vi "nipkg-updateControlFileMetadataField.vi"(0 "Package data":T1, 5 "Metadata field name":string, 7 "Metadata field index":u8, 9 "Metadata field value":string, 11 "error in (no error)":errorcluster) -> (4 "Package data out":T1, 15 "error out":errorcluster)   [LabVIEW 2014, in "nipkg-build-system.lvlib"]
uses:
  nipkg-build-system.lvlib
  types/Package data.ctl
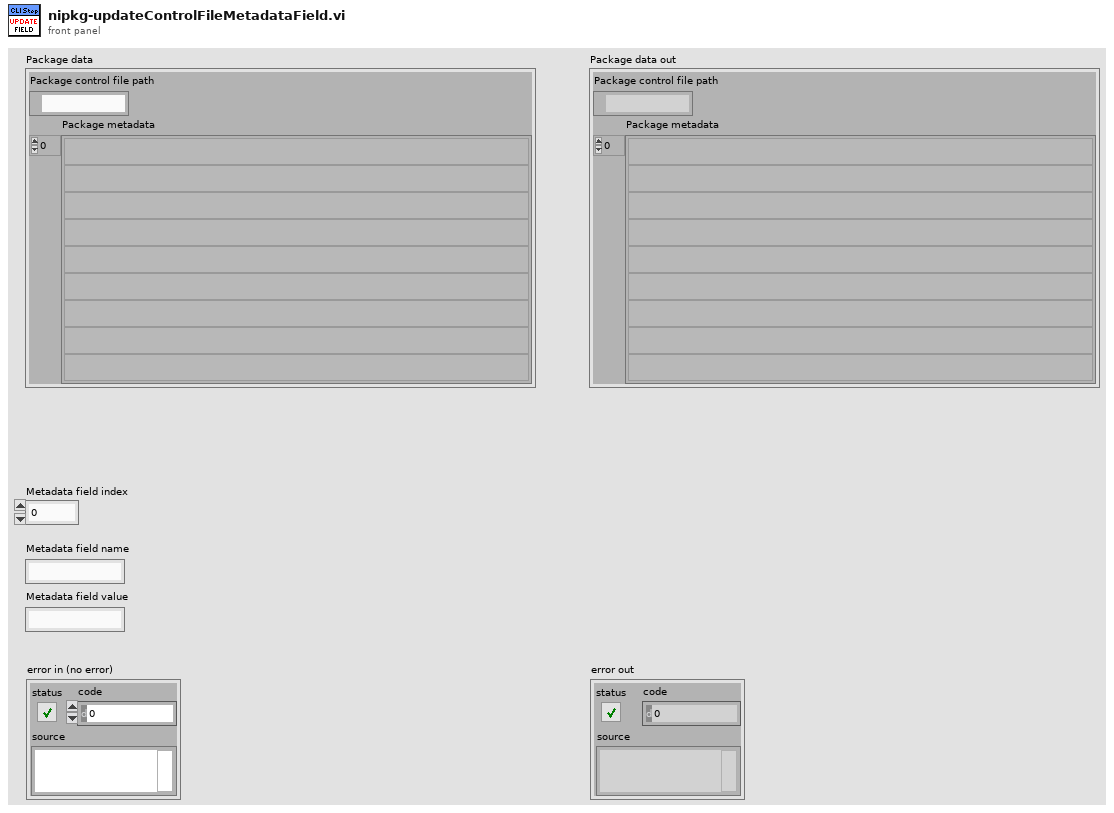
[diagram p1: front panel]
types:
  T1 = typedef "nipkg-build-system.lvlib/Package data.ctl" = cluster{"Package control file path":path, "Package metadata":string[]}
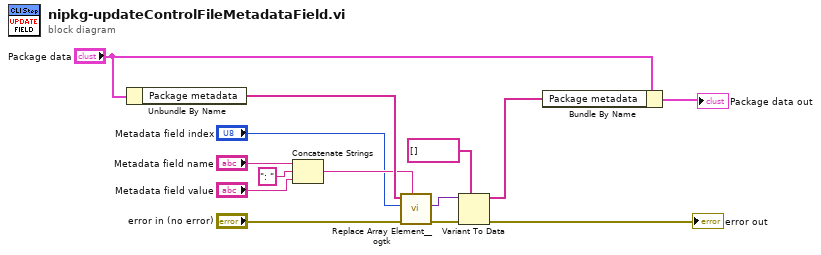
[diagram p0: block diagram]
diagram:
  n1 = Unbundle By Name("Package data") -> ("Package metadata"=w11:string[])
  n2 = Concatenate Strings("Metadata field name", ": " ("string"), "Metadata field value") -> (w10:string)
  n3 = call <userlib>:"Replace Array Element__ogtk.vi"("New Element"=w10, "error in (no error)"="error in (no error)", "Index (1D)"="Metadata field index", "MultiD Array"=w11) -> ("error out"=w6:errorcluster, "VMultiD Array"=w5:variant)  [unwired: 6 in]
  n4 = Variant To Data(error in=w6, type=string[] [], Variant=w5) -> (data=w3:string[], error out=→"error out":errorcluster)
  n5 = Bundle By Name(cluster="Package data", "Package metadata"=w3) -> (→"Package data out":T1)
